vi "create_pb_arrayofarrays_expansion_v2.vi"(0 "Arbitrary Waveform Array of Channels":T2(array[cluster])=[[{"AC Frequency (kHz)"=40.0, " Initial AC Ampl. (p-p/2)"=0.0, "Final AC Ampl."=0.0, "Initial DC Value"=-0.25, "Final DC Value"=0.05, "Constant"=165.3, "Gamma AC"=1.0, "String"="Channel 0 A", "Gamma DC"=1.0}, {"AC Frequency (kHz)"=40.0, " Initial AC Ampl. (p-p/2)"=0.0, "Final AC Ampl."=0.0, "Initial DC Value"=0.0, "Final DC Value"=0.0, "Constant"=165.2, "Gamma AC"=1.0, "String"="Channel 0 B", "Gamma DC"=1.0}, {"AC Frequency (kHz)"=40.0, " Initial AC Ampl. (p-p/2)"=0.0, "Final AC Ampl."=0.0, "Initial DC Value"=0.0, "Final DC Value"=0.0, "Constant"=163.20000000000002, "Gamma AC"=1.0, "String"="Channel 0 C", "Gamma DC"=1.0}], [{"AC Frequency (kHz)"=10.0, " Initial AC Ampl. (p-p/2)"=5.0, "Final AC Ampl."=0.0, "Initial DC Value"=0.2, "Final DC Value"=0.14, "Constant"=0.25, "Gamma AC"=1.0, "String"="Channel 1 A", "Gamma DC"=1.0}, {"AC Frequency (kHz)"=10.0, " Initial AC Ampl. (p-p/2)"=5.0, "Final AC Ampl."=0.0, "Initial DC Value"=0.1, "Final DC Value"=0.1, "Constant"=0.25, "Gamma AC"=1.0, "String"="Channel 1 B", "Gamma DC"=1.0}, {"AC Frequency (kHz)"=10.0, " Initial AC Ampl. (p-p/2)"=0.0, "Final AC Ampl."=0.0, "Initial DC Value"=0.0, "Final DC Value"=0.0, "Constant"=0.25, "Gamma AC"=1.0, "String"="Channel 1 C", "Gamma DC"=1.0}], [{"AC Frequency (kHz)"=10.0, " Initial AC Ampl. (p-p/2)"=0.0, "Final AC Ampl."=0.0, "Initial DC Value"=0.007, "Final DC Value"=0.04, "Constant"=0.0, "Gamma AC"=1.0, "String"="Channel 2 A", "Gamma DC"=1.0}, {"AC Frequency (kHz)"=10.0, " Initial AC Ampl. (p-p/2)"=0.0, "Final AC Ampl."=0.0, "Initial DC Value"=0.5, "Final DC Value"=0.5, "Constant"=0.0, "Gamma AC"=1.0, "String"="Channel 2 B", "Gamma DC"=1.0}, {"AC Frequency (kHz)"=10.0, " Initial AC Ampl. (p-p/2)"=0.0, "Final AC Ampl."=0.0, "Initial DC Value"=0.0, "Final DC Value"=0.0, "Constant"=0.0, "Gamma AC"=1.0, "String"="Channel 2 C", "Gamma DC"=1.0}], [{"AC Frequency (kHz)"=10.0, " Initial AC Ampl. (p-p/2)"=0.0, "Final AC Ampl."=0.0, "Initial DC Value"=1.0, "Final DC Value"=1.0, "Constant"=199.2, "Gamma AC"=1.0, "String"="Channel 3 A", "Gamma DC"=1.0}, {"AC Frequency (kHz)"=10.0, " Initial AC Ampl. (p-p/2)"=0.0, "Final AC Ampl."=0.0, "Initial DC Value"=1.0, "Final DC Value"=1.0, "Constant"=199.2, "Gamma AC"=1.0, "String"="Channel 3 B", "Gamma DC"=1.0}, {"AC Frequency (kHz)"=10.0, " Initial AC Ampl. (p-p/2)"=0.0, "Final AC Ampl."=0.0, "Initial DC Value"=1.0, "Final DC Value"=1.0, "Constant"=199.2, "Gamma AC"=1.0, "String"="Channel 3 C", "Gamma DC"=1.0}], [{"AC Frequency (kHz)"=10.0, " Initial AC Ampl. (p-p/2)"=0.0, "Final AC Ampl."=0.0, "Initial DC Value"=-0.1, "Final DC Value"=-0.04, "Constant"=199.2, "Gamma AC"=1.0, "String"="Channel 4 A", "Gamma DC"=1.0}, {"AC Frequency (kHz)"=10.0, " Initial AC Ampl. (p-p/2)"=0.0, "Final AC Ampl."=0.0, "Initial DC Value"=-0.1, "Final DC Value"=-0.04, "Constant"=199.2, "Gamma AC"=1.0, "String"="Channel 4 B", "Gamma DC"=1.0}, {"AC Frequency (kHz)"=10.0, " Initial AC Ampl. (p-p/2)"=0.0, "Final AC Ampl."=0.0, "Initial DC Value"=-0.1, "Final DC Value"=-0.04, "Constant"=199.2, "Gamma AC"=1.0, "String"="Channel 4 C", "Gamma DC"=1.0}], [{"AC Frequency (kHz)"=10.0, " Initial AC Ampl. (p-p/2)"=0.0, "Final AC Ampl."=0.0, "Initial DC Value"=-0.1, "Final DC Value"=-0.04, "Constant"=199.2, "Gamma AC"=1.0, "String"="Channel 5 A", "Gamma DC"=1.0}, {"AC Frequency (kHz)"=10.0, " Initial AC Ampl. (p-p/2)"=0.0, "Final AC Ampl."=0.0, "Initial DC Value"=-0.1, "Final DC Value"=-0.04, "Constant"=199.2, "Gamma AC"=1.0, "String"="Channel 5 B", "Gamma DC"=1.0}, {"AC Frequency (kHz)"=10.0, " Initial AC Ampl. (p-p/2)"=0.0, "Final AC Ampl."=0.0, "Initial DC Value"=-0.1, "Final DC Value"=-0.04, "Constant"=199.2, "Gamma AC"=1.0, "String"="Channel 5 C", "Gamma DC"=1.0}], [{"AC Frequency (kHz)"=10.0, " Initial AC Ampl. (p-p/2)"=0.0, "Final AC Ampl."=0.0, "Initial DC Value"=-0.1, "Final DC Value"=-0.04, "Constant"=199.2, "Gamma AC"=1.0, "String"="Channel 6 A", "Gamma DC"=1.0}, {"AC Frequency (kHz)"=10.0, " Initial AC Ampl. (p-p/2)"=0.0, "Final AC Ampl."=0.0, "Initial DC Value"=-0.1, "Final DC Value"=-0.04, "Constant"=199.2, "Gamma AC"=1.0, "String"="Channel 6 B", "Gamma DC"=1.0}, {"AC Frequency (kHz)"=10.0, " Initial AC Ampl. (p-p/2)"=0.0, "Final AC Ampl."=0.0, "Initial DC Value"=-0.1, "Final DC Value"=-0.04, "Constant"=199.2, "Gamma AC"=1.0, "String"="Channel 6 C", "Gamma DC"=1.0}], [{"AC Frequency (kHz)"=10.0, " Initial AC Ampl. (p-p/2)"=0.0, "Final AC Ampl."=0.0, "Initial DC Value"=-0.1, "Final DC Value"=-0.04, "Constant"=199.2, "Gamma AC"=1.0, "String"="Channel 7 A", "Gamma DC"=1.0}, {"AC Frequency (kHz)"=10.0, " Initial AC Ampl. (p-p/2)"=0.0, "Final AC Ampl."=0.0, "Initial DC Value"=-0.1, "Final DC Value"=-0.04, "Constant"=199.2, "Gamma AC"=1.0, "String"="Channel 7 B", "Gamma DC"=1.0}, {"AC Frequency (kHz)"=10.0, " Initial AC Ampl. (p-p/2)"=0.0, "Final AC Ampl."=0.0, "Initial DC Value"=-0.1, "Final DC Value"=-0.04, "Constant"=199.2, "Gamma AC"=1.0, "String"="Channel 7 C", "Gamma DC"=1.0}]] {"Gamma DC" format="%.2f"; "Gamma AC" format="%.2f"; "Constant" min=0.0 max=240.0 format="%.3f"; "Final DC Value" format="%.3f"; "Initial DC Value" format="%.3f"; "Final AC Ampl." format="%.3f"; "Initial AC Ampl. (p-p/2)" format="%.3f"; "AC Frequency (kHz)" format="%.2f"}, 2 "Parameters to Change":T9={"PB parameter to change"=0, "Column of\nData to Change\n(0, 1, 2, ....)"=0, "Column of\nDelay to Change\n(0, 1, 2, ....)"=11, "6713 DAC Ch\nto Change"=7, "column for waveform\n(red mot cooling)"=10, "# of PB arrays"=1, "column for waveform\n(dipole trap loading)"=10, "Power\nSupply\nChannel"=1} {"Power\nSupply\nChannel" min=1 max=2; "PB parameter to change" min=0 max=4}, 5 "87Sr Waveform Change Parameters":T6={"Channel to Change"=0, "Interval to Change"=1, "Waveform Parameter\nto Change"=8} {"Waveform Parameter\nto Change" items=["Constant", "Initial DC", "Final DC", "Gamma DC", "AC Frequency", "Initial AC", "Gamma AC", "Final AC", "Interval Length"]; "Interval to Change" items=["A", "B", "C", "D"]}, 7 "87Sr Interval Lengths (ms)":dbl[](array[numeric])=[55.0, 45.0, 1.0] format="%.3f", 9 "87Sr Intervals: ON or OFF?":bool[](array[boolean])=[TRUE, FALSE, FALSE], 11 "Generated Array":T7={"Step Size"=-0.03, "Use generated\nDAC array values?"=FALSE, "Number of DAC Array\nValues to Generate"=67, "Initial Value for DAC"=[1.0]} {"Initial Value for DAC" format="%.2f"; "Step Size" format="%.4f"}, 12 "Logarithmic Array":T5={"Initial Value"=1, "Fineness Factor"=1, "Number of Values"=10, "Generate Logarithmic\nArray?"=FALSE}, 13 "Lattice Waveform Array of Channels":T2(array[cluster])=[[{"AC Frequency (kHz)"=40.0, " Initial AC Ampl. (p-p/2)"=0.0, "Final AC Ampl."=0.0, "Initial DC Value"=-0.25, "Final DC Value"=0.05, "Constant"=165.3, "Gamma AC"=1.0, "String"="Channel 0 A", "Gamma DC"=1.0}, {"AC Frequency (kHz)"=40.0, " Initial AC Ampl. (p-p/2)"=0.0, "Final AC Ampl."=0.0, "Initial DC Value"=0.0, "Final DC Value"=0.0, "Constant"=165.2, "Gamma AC"=1.0, "String"="Channel 0 B", "Gamma DC"=1.0}, {"AC Frequency (kHz)"=40.0, " Initial AC Ampl. (p-p/2)"=0.0, "Final AC Ampl."=0.0, "Initial DC Value"=0.0, "Final DC Value"=0.0, "Constant"=163.20000000000002, "Gamma AC"=1.0, "String"="Channel 0 C", "Gamma DC"=1.0}], [{"AC Frequency (kHz)"=10.0, " Initial AC Ampl. (p-p/2)"=5.0, "Final AC Ampl."=0.0, "Initial DC Value"=0.2, "Final DC Value"=0.14, "Constant"=0.25, "Gamma AC"=1.0, "String"="Channel 1 A", "Gamma DC"=1.0}, {"AC Frequency (kHz)"=10.0, " Initial AC Ampl. (p-p/2)"=5.0, "Final AC Ampl."=0.0, "Initial DC Value"=0.1, "Final DC Value"=0.1, "Constant"=0.25, "Gamma AC"=1.0, "String"="Channel 1 B", "Gamma DC"=1.0}, {"AC Frequency (kHz)"=10.0, " Initial AC Ampl. (p-p/2)"=0.0, "Final AC Ampl."=0.0, "Initial DC Value"=0.0, "Final DC Value"=0.0, "Constant"=0.25, "Gamma AC"=1.0, "String"="Channel 1 C", "Gamma DC"=1.0}], [{"AC Frequency (kHz)"=10.0, " Initial AC Ampl. (p-p/2)"=0.0, "Final AC Ampl."=0.0, "Initial DC Value"=0.007, "Final DC Value"=0.04, "Constant"=0.0, "Gamma AC"=1.0, "String"="Channel 2 A", "Gamma DC"=1.0}, {"AC Frequency (kHz)"=10.0, " Initial AC Ampl. (p-p/2)"=0.0, "Final AC Ampl."=0.0, "Initial DC Value"=0.5, "Final DC Value"=0.5, "Constant"=0.0, "Gamma AC"=1.0, "String"="Channel 2 B", "Gamma DC"=1.0}, {"AC Frequency (kHz)"=10.0, " Initial AC Ampl. (p-p/2)"=0.0, "Final AC Ampl."=0.0, "Initial DC Value"=0.0, "Final DC Value"=0.0, "Constant"=0.0, "Gamma AC"=1.0, "String"="Channel 2 C", "Gamma DC"=1.0}], [{"AC Frequency (kHz)"=10.0, " Initial AC Ampl. (p-p/2)"=0.0, "Final AC Ampl."=0.0, "Initial DC Value"=1.0, "Final DC Value"=1.0, "Constant"=199.2, "Gamma AC"=1.0, "String"="Channel 3 A", "Gamma DC"=1.0}, {"AC Frequency (kHz)"=10.0, " Initial AC Ampl. (p-p/2)"=0.0, "Final AC Ampl."=0.0, "Initial DC Value"=1.0, "Final DC Value"=1.0, "Constant"=199.2, "Gamma AC"=1.0, "String"="Channel 3 B", "Gamma DC"=1.0}, {"AC Frequency (kHz)"=10.0, " Initial AC Ampl. (p-p/2)"=0.0, "Final AC Ampl."=0.0, "Initial DC Value"=1.0, "Final DC Value"=1.0, "Constant"=199.2, "Gamma AC"=1.0, "String"="Channel 3 C", "Gamma DC"=1.0}], [{"AC Frequency (kHz)"=10.0, " Initial AC Ampl. (p-p/2)"=0.0, "Final AC Ampl."=0.0, "Initial DC Value"=-0.1, "Final DC Value"=-0.04, "Constant"=199.2, "Gamma AC"=1.0, "String"="Channel 4 A", "Gamma DC"=1.0}, {"AC Frequency (kHz)"=10.0, " Initial AC Ampl. (p-p/2)"=0.0, "Final AC Ampl."=0.0, "Initial DC Value"=-0.1, "Final DC Value"=-0.04, "Constant"=199.2, "Gamma AC"=1.0, "String"="Channel 4 B", "Gamma DC"=1.0}, {"AC Frequency (kHz)"=10.0, " Initial AC Ampl. (p-p/2)"=0.0, "Final AC Ampl."=0.0, "Initial DC Value"=-0.1, "Final DC Value"=-0.04, "Constant"=199.2, "Gamma AC"=1.0, "String"="Channel 4 C", "Gamma DC"=1.0}], [{"AC Frequency (kHz)"=10.0, " Initial AC Ampl. (p-p/2)"=0.0, "Final AC Ampl."=0.0, "Initial DC Value"=-0.1, "Final DC Value"=-0.04, "Constant"=199.2, "Gamma AC"=1.0, "String"="Channel 5 A", "Gamma DC"=1.0}, {"AC Frequency (kHz)"=10.0, " Initial AC Ampl. (p-p/2)"=0.0, "Final AC Ampl."=0.0, "Initial DC Value"=-0.1, "Final DC Value"=-0.04, "Constant"=199.2, "Gamma AC"=1.0, "String"="Channel 5 B", "Gamma DC"=1.0}, {"AC Frequency (kHz)"=10.0, " Initial AC Ampl. (p-p/2)"=0.0, "Final AC Ampl."=0.0, "Initial DC Value"=-0.1, "Final DC Value"=-0.04, "Constant"=199.2, "Gamma AC"=1.0, "String"="Channel 5 C", "Gamma DC"=1.0}], [{"AC Frequency (kHz)"=10.0, " Initial AC Ampl. (p-p/2)"=0.0, "Final AC Ampl."=0.0, "Initial DC Value"=-0.1, "Final DC Value"=-0.04, "Constant"=199.2, "Gamma AC"=1.0, "String"="Channel 6 A", "Gamma DC"=1.0}, {"AC Frequency (kHz)"=10.0, " Initial AC Ampl. (p-p/2)"=0.0, "Final AC Ampl."=0.0, "Initial DC Value"=-0.1, "Final DC Value"=-0.04, "Constant"=199.2, "Gamma AC"=1.0, "String"="Channel 6 B", "Gamma DC"=1.0}, {"AC Frequency (kHz)"=10.0, " Initial AC Ampl. (p-p/2)"=0.0, "Final AC Ampl."=0.0, "Initial DC Value"=-0.1, "Final DC Value"=-0.04, "Constant"=199.2, "Gamma AC"=1.0, "String"="Channel 6 C", "Gamma DC"=1.0}], [{"AC Frequency (kHz)"=10.0, " Initial AC Ampl. (p-p/2)"=0.0, "Final AC Ampl."=0.0, "Initial DC Value"=-0.1, "Final DC Value"=-0.04, "Constant"=199.2, "Gamma AC"=1.0, "String"="Channel 7 A", "Gamma DC"=1.0}, {"AC Frequency (kHz)"=10.0, " Initial AC Ampl. (p-p/2)"=0.0, "Final AC Ampl."=0.0, "Initial DC Value"=-0.1, "Final DC Value"=-0.04, "Constant"=199.2, "Gamma AC"=1.0, "String"="Channel 7 B", "Gamma DC"=1.0}, {"AC Frequency (kHz)"=10.0, " Initial AC Ampl. (p-p/2)"=0.0, "Final AC Ampl."=0.0, "Initial DC Value"=-0.1, "Final DC Value"=-0.04, "Constant"=199.2, "Gamma AC"=1.0, "String"="Channel 7 C", "Gamma DC"=1.0}]] {"Gamma DC" format="%.2f"; "Gamma AC" format="%.2f"; "Constant" min=0.0 max=240.0 format="%.3f"; "Final DC Value" format="%.3f"; "Initial DC Value" format="%.3f"; "Final AC Ampl." format="%.3f"; "Initial AC Ampl. (p-p/2)" format="%.3f"; "AC Frequency (kHz)" format="%.2f"}) -> (1 "changed\nquantity":dbl[](array[numeric]), 4 "Lattice Waveform \nArray of Channels":T1(array[cluster]), 6 "87 Sr ArbWaveform \nArray of Channels":T1(array[cluster]), 8 "87Sr ArbWaveform Interval Lengths":dbl[][](array[numeric]), 10 "Generated\nDAC Array":dbl[](array[numeric])=[1.0, 0.97, 0.94, 0.9099999999999999, 0.8799999999999999, 0.8499999999999999, 0.8199999999999998, 0.7899999999999998, 0.7599999999999998, 0.7299999999999998, 0.6999999999999997, 0.6699999999999997, 0.6399999999999997, 0.6099999999999997, 0.5799999999999996, 0.5499999999999996, 0.5199999999999996, 0.48999999999999955, 0.4599999999999995, 0.4299999999999995, 0.39999999999999947, 0.36999999999999944, 0.3399999999999994, 0.3099999999999994, 0.27999999999999936, 0.24999999999999936, 0.21999999999999936, 0.18999999999999936, 0.15999999999999936, 0.12999999999999937, 0.09999999999999937, 0.06999999999999937, 0.03999999999999937, 0.00999999999999937, -0.02000000000000063, -0.05000000000000063, -0.08000000000000063, -0.11000000000000063, -0.14000000000000062, -0.17000000000000062, -0.20000000000000062, -0.23000000000000062, -0.2600000000000006, -0.2900000000000006, -0.3200000000000006, -0.35000000000000064, -0.38000000000000067, -0.4100000000000007, -0.4400000000000007, -0.47000000000000075, -0.5000000000000008, -0.5300000000000008, -0.5600000000000008, -0.5900000000000009, -0.6200000000000009, -0.6500000000000009, -0.6800000000000009, -0.710000000000001, -0.740000000000001, -0.770000000000001, -0.800000000000001, -0.8300000000000011, -0.8600000000000011, -0.8900000000000011, -0.9200000000000012, -0.9500000000000012, -0.9800000000000012, -1.0100000000000011] format="%.4f", 15 "output params to change":T8)   [LabVIEW 2013]
panel:
  in  "Case Constant\n(See Context Help)":bool
  out "PB Array of Arrays":T3(array[cluster])
  in  "PulseBlaster Array of Arrays":T4(array[cluster])=[{"Data Field"=0, "Delay"=0.005, "OP code"=8, "Output Bits"=[FALSE, TRUE, FALSE, FALSE, FALSE, FALSE, FALSE, FALSE, FALSE, FALSE, FALSE, FALSE, TRUE, FALSE, FALSE, FALSE, FALSE, FALSE, FALSE, FALSE, FALSE, FALSE, FALSE, FALSE], "String"="cool mot coils"}, {"Data Field"=300, "Delay"=0.000999, "OP code"=2, "Output Bits"=[TRUE, TRUE, TRUE, TRUE, FALSE, FALSE, TRUE, FALSE, FALSE, TRUE, FALSE, FALSE, TRUE, TRUE, FALSE, TRUE, TRUE, FALSE, FALSE, FALSE, FALSE, FALSE, FALSE, FALSE], "String"="mot load loop"}, {"Data Field"=1, "Delay"=1e-06, "OP code"=3, "Output Bits"=[TRUE, TRUE, TRUE, TRUE, FALSE, FALSE, TRUE, FALSE, FALSE, TRUE, FALSE, FALSE, TRUE, TRUE, FALSE, TRUE, TRUE, FALSE, FALSE, FALSE, FALSE, FALSE, FALSE, FALSE, FALSE], "String"=""}, {"Data Field"=0, "Delay"=0.001, "OP code"=0, "Output Bits"=[TRUE, TRUE, TRUE, TRUE, FALSE, FALSE, TRUE, FALSE, FALSE, TRUE, FALSE, FALSE, TRUE, TRUE, FALSE, TRUE, TRUE, FALSE, FALSE, FALSE, FALSE, FALSE, FALSE, FALSE], "String"=""}, {"Data Field"=2, "Delay"=0.000999, "OP code"=2, "Output Bits"=[TRUE, TRUE, TRUE, TRUE, FALSE, FALSE, TRUE, FALSE, FALSE, TRUE, FALSE, FALSE, TRUE, TRUE, FALSE, TRUE, TRUE, FALSE, FALSE, FALSE, FALSE, FALSE, FALSE, FALSE], "String"="mot decay loop"}, {"Data Field"=4, "Delay"=1e-06, "OP code"=3, "Output Bits"=[TRUE, TRUE, TRUE, TRUE, FALSE, FALSE, TRUE, FALSE, FALSE, TRUE, FALSE, FALSE, TRUE, TRUE, FALSE, TRUE, TRUE, FALSE, FALSE, FALSE, FALSE, FALSE, FALSE, FALSE], "String"=""}, {"Data Field"=0, "Delay"=0.000908, "OP code"=0, "Output Bits"=[TRUE, TRUE, TRUE, TRUE, FALSE, FALSE, TRUE, FALSE, FALSE, TRUE, FALSE, FALSE, TRUE, TRUE, FALSE, TRUE, TRUE, FALSE, FALSE, FALSE, FALSE, FALSE, FALSE, FALSE], "String"=""}, {"Data Field"=0, "Delay"=0.00865, "OP code"=0, "Output Bits"=[TRUE, TRUE, TRUE, TRUE, FALSE, FALSE, TRUE, FALSE, FALSE, TRUE, FALSE, FALSE, TRUE, TRUE, FALSE, TRUE, TRUE, FALSE, FALSE, FALSE, FALSE, FALSE, FALSE, FALSE], "String"=""}, {"Data Field"=0, "Delay"=0.004, "OP code"=0, "Output Bits"=[TRUE, TRUE, FALSE, TRUE, FALSE, FALSE, TRUE, FALSE, FALSE, TRUE, FALSE, FALSE, TRUE, TRUE, FALSE, TRUE, TRUE, FALSE, FALSE, FALSE, FALSE, FALSE, FALSE, FALSE], "String"=""}, {"Data Field"=0, "Delay"=0.0045, "OP code"=0, "Output Bits"=[TRUE, TRUE, FALSE, TRUE, FALSE, FALSE, TRUE, FALSE, FALSE, TRUE, FALSE, FALSE, TRUE, FALSE, FALSE, FALSE, TRUE, FALSE, FALSE, FALSE, FALSE, FALSE, FALSE, FALSE], "String"="Blue MOT Cooling Time"}, {"Data Field"=0, "Delay"=0.05, "OP code"=0, "Output Bits"=[FALSE, TRUE, FALSE, FALSE, FALSE, FALSE, FALSE, FALSE, FALSE, TRUE, TRUE, FALSE, TRUE, FALSE, FALSE, FALSE, FALSE, FALSE, FALSE, FALSE, FALSE, FALSE, FALSE, FALSE], "String"="Red MOT Cooling Time =="}, {"Data Field"=0, "Delay"=0.01, "OP code"=0, "Output Bits"=[FALSE, TRUE, FALSE, FALSE, FALSE, FALSE, FALSE, FALSE, FALSE, FALSE, FALSE, FALSE, FALSE, FALSE, FALSE, FALSE, FALSE, FALSE, FALSE, FALSE, FALSE, FALSE, FALSE, FALSE], "String"="PAS Beam with RED MOT            DELAY TIME BEFORE INTERAC"}, {"Data Field"=0, "Delay"=0.005, "OP code"=0, "Output Bits"=[FALSE, TRUE, FALSE, FALSE, FALSE, FALSE, FALSE, FALSE, FALSE, FALSE, FALSE, FALSE, FALSE, FALSE, FALSE, FALSE, TRUE, FALSE, FALSE, FALSE, FALSE, FALSE, FALSE, FALSE], "String"="image 12 delay (150n=90ndelay) INTERAC TIME"}, {"Data Field"=0, "Delay"=5e-05, "OP code"=0, "Output Bits"=[FALSE, TRUE, FALSE, FALSE, FALSE, FALSE, FALSE, FALSE, FALSE, FALSE, FALSE, FALSE, FALSE, FALSE, FALSE, FALSE, TRUE, TRUE, FALSE, FALSE, FALSE, FALSE, FALSE, FALSE], "String"="image beam on"}, {"Data Field"=0, "Delay"=0.0002, "OP code"=0, "Output Bits"=[FALSE, FALSE, FALSE, FALSE, FALSE, TRUE, FALSE, FALSE, FALSE, FALSE, FALSE, FALSE, FALSE, FALSE, FALSE, FALSE, TRUE, TRUE, FALSE, FALSE, FALSE, FALSE, FALSE, FALSE], "String"="camera minimum exposure time"}, {"Data Field"=0, "Delay"=0.07, "OP code"=0, "Output Bits"=[FALSE, FALSE, FALSE, FALSE, FALSE, FALSE, FALSE, FALSE, FALSE, FALSE, FALSE, FALSE, FALSE, FALSE, FALSE, FALSE, FALSE, TRUE, FALSE, FALSE, FALSE, FALSE, FALSE, FALSE], "String"="PixelFly Readout 1"}, {"Data Field"=0, "Delay"=0.005, "OP code"=0, "Output Bits"=[FALSE, FALSE, FALSE, FALSE, FALSE, FALSE, FALSE, FALSE, FALSE, FALSE, FALSE, FALSE, FALSE, FALSE, FALSE, FALSE, TRUE, TRUE, FALSE, FALSE, FALSE, FALSE, FALSE, FALSE], "String"="shutter opening time"}, {"Data Field"=0, "Delay"=0.0002, "OP code"=0, "Output Bits"=[FALSE, FALSE, FALSE, FALSE, FALSE, TRUE, FALSE, FALSE, FALSE, FALSE, FALSE, FALSE, FALSE, FALSE, FALSE, FALSE, TRUE, TRUE, FALSE, FALSE, FALSE, FALSE, FALSE, FALSE], "String"="Pixelfly exposure 2"}, {"Data Field"=0, "Delay"=0.07, "OP code"=0, "Output Bits"=[FALSE, FALSE, FALSE, FALSE, FALSE, FALSE, FALSE, FALSE, FALSE, FALSE, FALSE, FALSE, FALSE, FALSE, FALSE, FALSE, FALSE, FALSE, FALSE, FALSE, FALSE, FALSE, FALSE, FALSE], "String"="PixelFly readout 2"}, {"Data Field"=0, "Delay"=0.001, "OP code"=6, "Output Bits"=[FALSE, TRUE, TRUE, TRUE, FALSE, FALSE, FALSE, FALSE, FALSE, FALSE, FALSE, FALSE, TRUE, TRUE, FALSE, TRUE, FALSE, FALSE, FALSE, FALSE, FALSE, FALSE, FALSE, FALSE], "String"=""}] {"OP code" items=["Continue", "Stop", "Loop", "End Loop", "Jump", "Return", "Go To", "Long Delay", "Wait"]; "Delay" format="%.3p"}
  in  "Manual Array":dbl[](array[numeric])=[0.05, 0.1, 0.15, 0.2, 0.25, 0.3, 0.35, 0.4, 0.45, 0.5, 9.6, 0.24, 0.26, 5.28, 0.3, 0.32, 0.34, 0.36, 0.38, 0.4, 5.0, 5.2, 5.4, 5.6, 5.8, 6.0, 6.2, 6.4, 6.6, 6.8, 7.0, 7.199999999999999, 7.4, 7.6, 7.800000000000001, 9.0, 6.8, 7.2, 7.6, 8.0, 8.4, 8.8, 9.0, 9.2, 9.4, 9.6, 9.8, 10.0, 0.4, 0.2, 0.0001, 0.0001, 0.0001, 0.0001, 0.0001, 0.0001, 0.0001, 0.0001, 0.0001, 0.0001, 0.0001, 0.0001, 0.0001, 0.0001, 0.0001, 0.0001, 0.0001, 0.0001, 0.0001, 0.0001, 0.0001, 0.0001, 0.0001, 0.0001, 0.0001, 0.0001, 0.0001, 0.0001, 0.0001, 0.0001, 0.0001, 0.0001, 0.0001, 0.0001, 0.0001, 0.0001, 0.0001, 0.0001, 0.0001, 0.0001, 0.0001, 0.0001, 0.0001, 0.0001, 0.0001, 0.0001, 0.0001, 0.0001, 0.0001, 0.0001, 0.0001, 0.0001, 0.0001, 0.0001, 0.0001, 0.0001, 0.0001, 0.0001, 0.0001, 0.0001, 0.0001, 0.0001, 0.0001, 0.0001, 0.0001, 0.0001, 0.0001, 0.0001, 0.0001, 0.0001, 0.0001, 0.0001, 0.0001, 0.0001, 0.0001, 0.0001, 0.0001, 0.0001, 0.0001, 0.0001, 0.0001, 0.0001, 0.0001, 0.0001, 0.0001, 0.0001, 0.0001, 0.0001, 0.0001, 0.0001, 0.0001, 0.0001, 0.0001, 0.0001, 0.0001, 0.0001, 0.0, 0.0, 0.0, 0.0, 0.0, 0.0, 0.0, 0.0, 0.0, 0.0, 0.0, 0.0, 0.0, 0.0, 0.0, 0.0, 0.0, 0.0, 0.0, 0.0, 0.0, 0.0, 0.0, 0.0, 0.0, 0.0, 0.0, 0.0, 0.0, 0.0, 0.0, 0.0, 0.0, 0.0, 0.0, 0.0, 0.0, 0.0, 0.0, 0.0, 0.0, 0.0, 0.0, 0.0, 0.0, 0.0, 0.0, 0.0, 0.0, 0.0, 0.0, 0.0, 0.0, 0.0, 0.0, 0.0, 0.0, 0.0, 0.0, 0.0, 0.0, 0.0, 0.0, 0.0, 0.0, 0.0, 0.0, 0.0, 0.0, 0.0, 0.0, 0.0, 0.0, 0.0, 0.0, 0.0, 0.0, 0.0, 0.0, 0.0, 0.0, 0.0, 0.0, 0.0, 0.0, 0.0, 0.0, 0.0, 0.0, 0.0, 0.0, 0.0, 0.0, 0.0, 0.0, 0.0, 0.0, 0.0, 0.0, 0.0, 0.0, 0.0, 0.0, 0.0, 0.0, 0.0, 0.0, 0.0, 0.0, 0.0, 0.0, 0.0, 0.0, 0.0, 0.0, 0.0, 0.0, 0.0, 0.0, 0.0, 0.0, 0.0, 0.0, 0.0, 0.0, 0.0, 0.0, 0.0, 0.0, 0.0, 0.0, 0.0, 0.0, 0.0, 0.0, 0.0, 0.0, 0.0, 0.0, 0.0, 0.0, 0.0, 0.0, 0.0, 0.0, 0.0, 0.0, 0.0, 0.0, 0.0, 0.0, 0.0, 0.0, 0.0, 0.0, 0.0, 0.0, 0.0, 0.0, 0.0, 0.0, 0.0, 0.0, 0.0, 0.0, 0.0, 0.0, 0.0, 0.0, 0.0, 0.0, 0.0, 0.0, 0.0, 0.0, 0.0, 0.0, 0.0, 0.0, 0.0, 0.0, 0.0, 0.0, 0.0, 0.0, 0.0, 0.0, 0.0, 0.0, 0.0, 0.0, 0.0, 0.0, 0.0, 0.0, 0.0, 0.0, 0.0, 0.0, 0.0, 0.0, 0.0, 0.0, 0.0, 0.0, 0.0, 0.0, 0.0, 0.0, 0.0, 0.0, 0.0, 0.0, 0.0, 0.0, 0.0, 0.0, 0.0, 0.0, 0.0, 0.0, 0.0, 0.0, 0.0, 0.0, 0.0, 0.0, 0.0, 0.0, 0.0, 0.0, 0.0, 0.0, 0.0, 0.0, 0.0, 0.0, 0.0, 0.0, 0.0, 0.0, 0.0, 0.0, 0.0, 0.0, 0.0, 0.0, 0.0, 0.0, 0.0, 0.0, 0.0, 0.0, 0.0, 0.0, 0.0, 0.0, 0.0, 0.0, 0.0, 0.0, 0.0, 0.0, 0.0, 0.0, 0.0, 0.0, 0.0, 0.0, 0.0, 0.0, 0.0, 0.0, 0.0, 0.0, 0.0, 0.0, 0.0, 0.0, 0.0, 0.0, 0.0, 0.0, 0.0, 0.0, 0.0, 0.0, 0.0, 0.0, 0.0, 0.0, 0.0, 0.0, 0.0, 0.0, 0.0, 0.0, 0.0, 0.0, 0.0, 0.0, 0.0, 0.0, 0.0, 0.0, 0.0, 0.0, 0.0, 0.0, 0.0, 0.0, 0.0, 0.0, 0.0, 0.0, 0.0, 0.0, 0.0, 0.0, 0.0, 0.0, 0.0, 0.0, 0.0, 0.0, 0.0, 0.0, 0.0, 0.0, 0.0, 0.0, 0.0, 0.0, 0.0, 0.0, 0.0, 0.0, 0.0, 0.0, 0.0, 0.0, 0.0, 0.0, 0.0, 0.0, 0.0, 0.0, 0.0, 0.0, 0.0, 0.0, 0.0, 0.0, 0.0, 0.0] caption="Manual array" format="%.3f"
  out "red mot cooling time":dbl[](array[numeric])
  # "(smaller makes\nblue)"
  # "(smaller makes\nblue)"
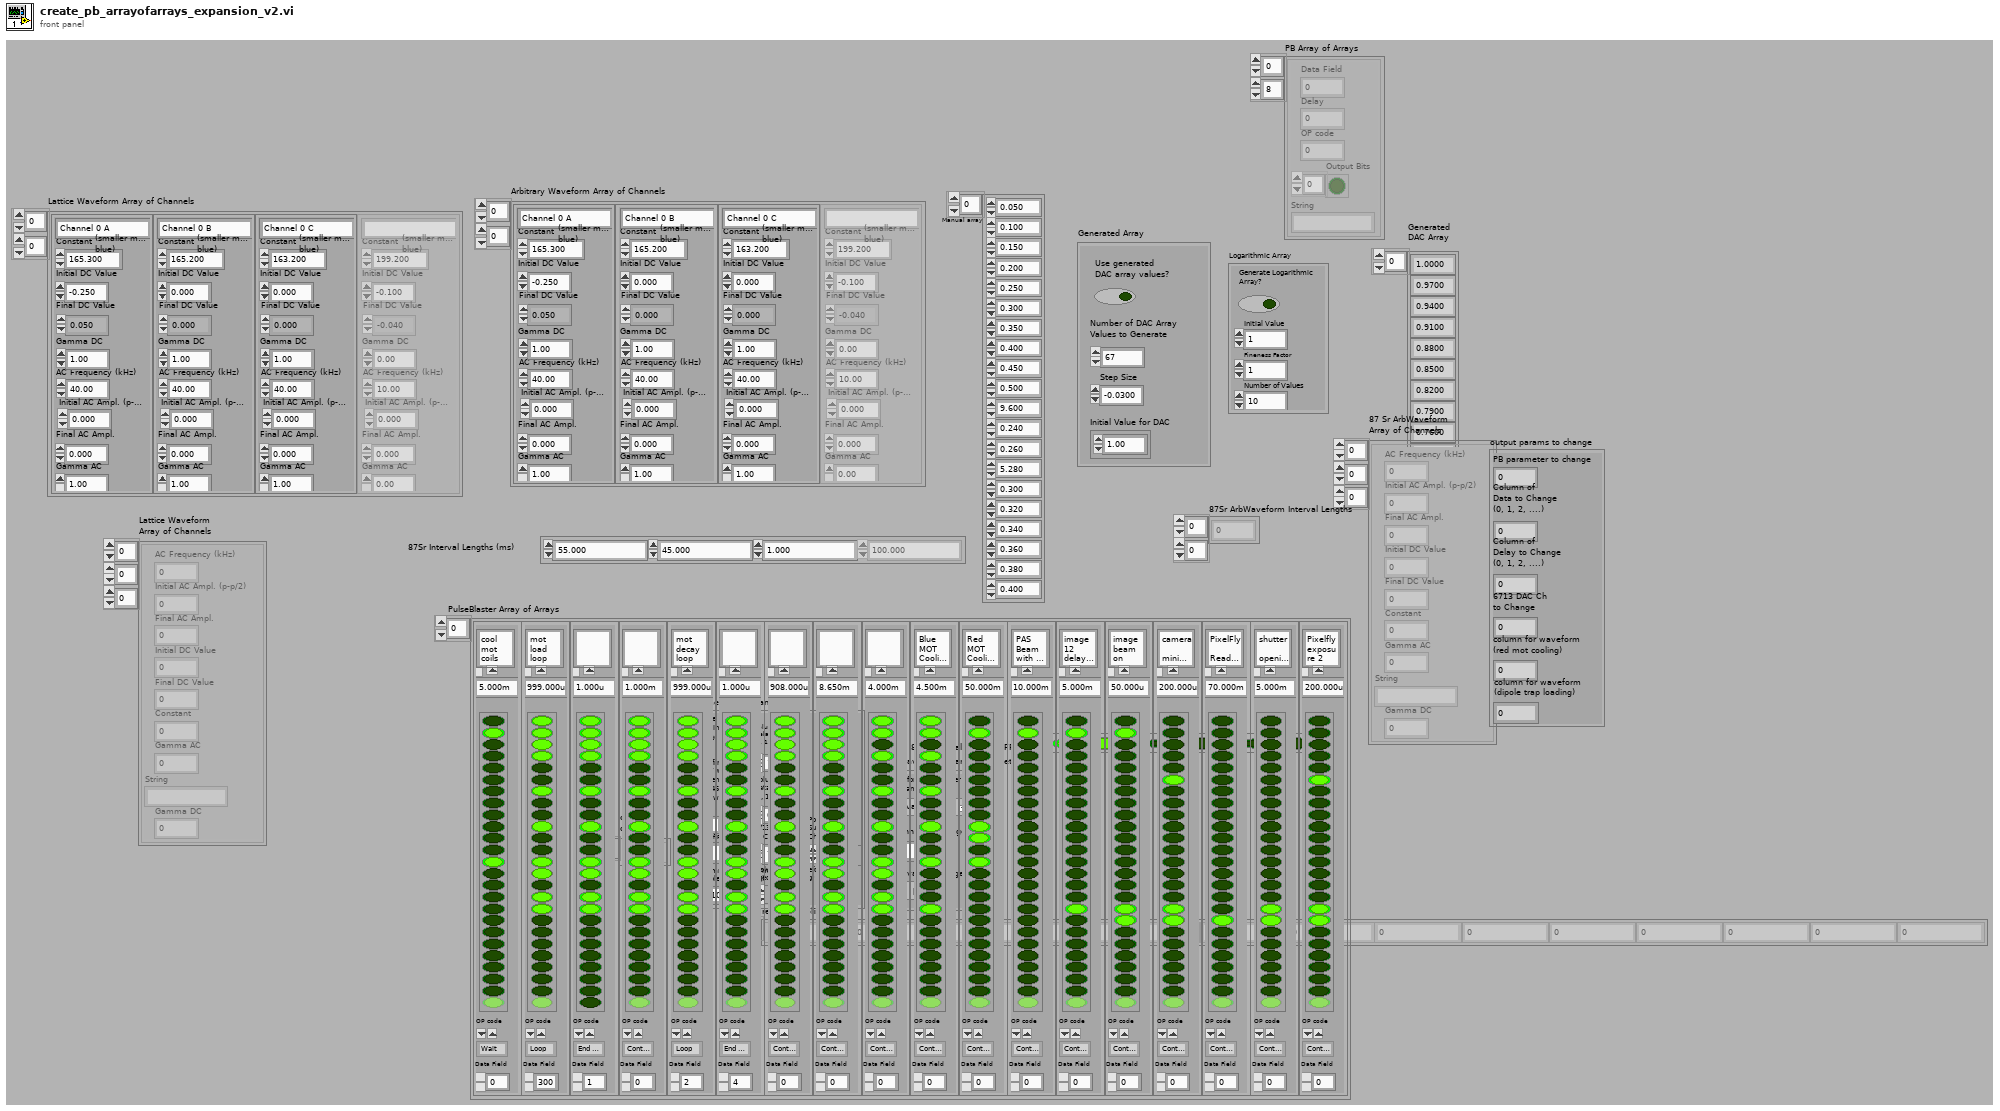
[diagram p1: front panel]
types:
  T1 = cluster{"AC Frequency (kHz)":dbl, "Initial AC Ampl. (p-p/2)":dbl, "Final AC Ampl.":dbl, "Initial DC Value":dbl, "Final DC Value":dbl, "Constant":dbl, "Gamma AC":dbl, "String":string, "Gamma DC":dbl}[][][]
  T2 = cluster{"AC Frequency (kHz)":dbl, " Initial AC Ampl. (p-p/2)":dbl, "Final AC Ampl.":dbl, "Initial DC Value":dbl, "Final DC Value":dbl, "Constant":dbl, "Gamma AC":dbl, "String":string, "Gamma DC":dbl}[][]
  T3 = cluster{"Data Field":u32, "Delay":dbl, "OP code":u8, "Output Bits":bool[], "String":string}[][]
  T4 = cluster{"Data Field":u32, "Delay":dbl, "OP code":u8, "Output Bits":bool[], "String":string}[]
  T5 = cluster{"Initial Value":i32, "Fineness Factor":i32, "Number of Values":i32, "Generate Logarithmic\nArray?":bool}
  T6 = cluster{"Channel to Change":i8, "Interval to Change":i8, "Waveform Parameter\nto Change":u16}
  T7 = cluster{"Step Size":dbl, "Use generated\nDAC array values?":bool, "Number of DAC Array\nValues to Generate":i32, "Initial Value for DAC":dbl[]}
  T8 = cluster{"PB parameter to change":i8, "Column of\nData to Change\n(0, 1, 2, ....)":i32, "Column of\nDelay to Change\n(0, 1, 2, ....)":i32, "6713 DAC Ch\nto Change":i32, "column for waveform\n(red mot cooling)":i32, "column for waveform\n(dipole trap loading)":i32}
  T9 = cluster{"PB parameter to change":i8, "Column of\nData to Change\n(0, 1, 2, ....)":i32, "Column of\nDelay to Change\n(0, 1, 2, ....)":i32, "6713 DAC Ch\nto Change":i32, "column for waveform\n(red mot cooling)":i32, "# of PB arrays":i32, "column for waveform\n(dipole trap loading)":i32, "Power\nSupply\nChannel":i32}
  T10 = cluster{"AC Frequency (kHz)":dbl, " Initial AC Ampl. (p-p/2)":dbl, "Final AC Ampl.":dbl, "Initial DC Value":dbl, "Final DC Value":dbl, "Constant":dbl, "Gamma AC":dbl, "String":string, "Gamma DC":dbl}
  T11 = cluster{"Data Field":u32, "Delay":dbl, "OP code":u8, "Output Bits":bool[], "String":string}
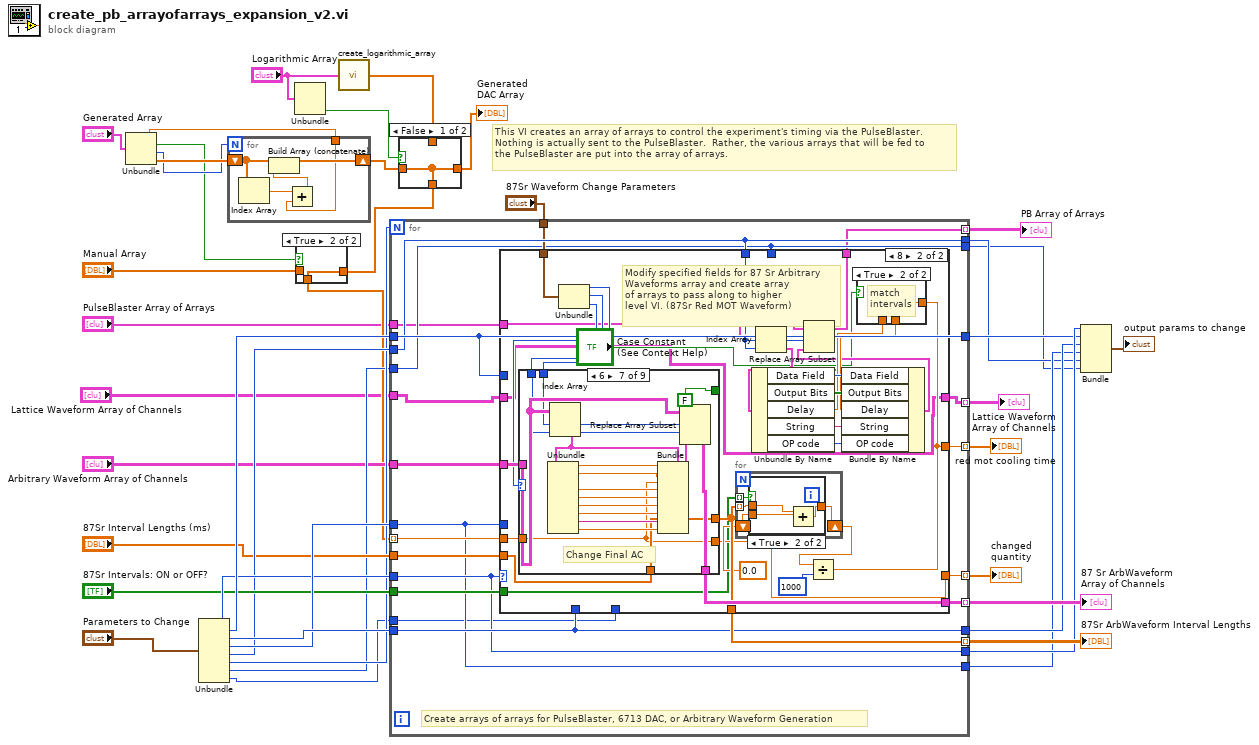
[diagram p0: block diagram]
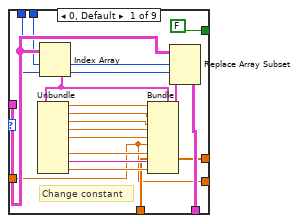
[diagram p7: hidden frame]
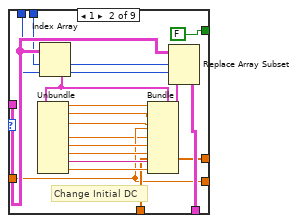
[diagram p8: hidden frame]
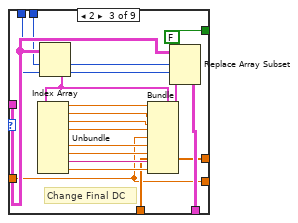
[diagram p9: hidden frame]
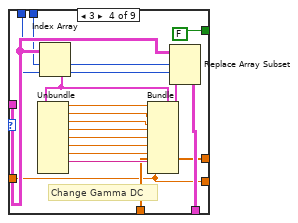
[diagram p10: hidden frame]
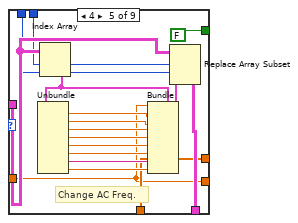
[diagram p11: hidden frame]
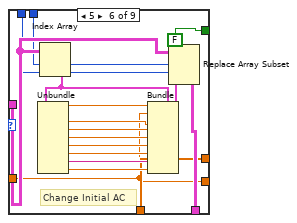
[diagram p12: hidden frame]
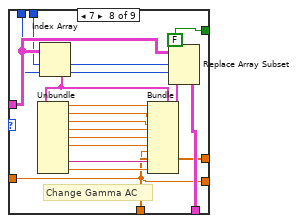
[diagram p13: hidden frame]
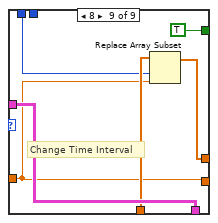
[diagram p14: hidden frame]
diagram:
  # "This VI creates an array of arrays to control the experiment's timing via the PulseBlaster.\nNothing is actually sent to the PulseBlaster.  Rather, the various arrays that will be fed to\nthe PulseBlaster are put into the array of arrays."
  n1 = Unbundle("Generated Array") -> ("Step Size"=w23:dbl, "Use generated\nDAC array values?"=w5:bool, "Number of DAC Array\nValues to Generate"=w24:i32, "Initial Value for DAC"=w25:dbl[])
  n2 = Unbundle("Parameters to Change") -> ("PB parameter to change"=w35:i8, "Column of\nData to Change\n(0, 1, 2, ....)"=w36:i32, "Column of\nDelay to Change\n(0, 1, 2, ....)"=w38:i32, "6713 DAC Ch\nto Change"=w37:i32, "column for waveform\n(red mot cooling)"=w29:i32, "# of PB arrays"=w19:i32, "column for waveform\n(dipole trap loading)"=w17:i32, "Power\nSupply\nChannel"=w15:i32)
  n3 = for {
    N: w24 -> [_]
    shift-right: [w47] -> w11
    shift-left: w25 -> [w46]
    tunnel: w23 -> [w42]
    i -> [w45]
    n4 = Index Array(array=w46, index=w45) -> (element=w44:dbl)
    n5 = Add(x=w44, y=w42) -> (x+y=w43:dbl)
    n6 = Build Array (concatenate)(w46, w43) -> (w47:dbl[])
  }
  n7 = Unbundle("Logarithmic Array") -> ("Generate Logarithmic\nArray?"=w12:bool)  [unwired: 3 out]
  n8 = call "create_logarithmic_array.vi"("Logarithmic Array"="Logarithmic Array") -> ("Generated Log Array"=w10:dbl[])
  n9 = case shown="False" w12 {
    tunnel: [w48 w49] -> w13
    tunnel: w11 -> [w48 _]
    tunnel: w10 -> [_ w49]
    tunnel: [w48 w49] -> w9
    frame False {
    }
    frame True {
    }
  }
  "Generated\nDAC Array" <- w13
  n10 = case shown="True" w5 {
    tunnel: w9 -> [_ w51]
    tunnel: "Manual Array" -> [w50 _]
    tunnel: [w50 w51] -> w6
    frame False {
    }
    frame True {
    }
  }
  n11 = for {
    N: w19 -> [_]
    tunnel: [w62] -> w32
    tunnel: w6 -> [w71] mode=indexing
    tunnel: "87Sr Intervals: ON or OFF?" -> [w70]
    tunnel: [w69] -> w41 mode=indexing
    tunnel: [w68] -> w40 mode=indexing
    tunnel: "Arbitrary Waveform Array of Channels" -> [w67]
    tunnel: w38 -> [w65]
    tunnel: w37 -> [w63]
    tunnel: w36 -> [w62]
    tunnel: w35 -> [w64]
    tunnel: "87Sr Interval Lengths (ms)" -> [w66]
    tunnel: [w65] -> w31
    tunnel: [w64] -> w33
    tunnel: [w63] -> w30
    tunnel: w29 -> [w61]
    tunnel: [w61] -> w28
    tunnel: [w60] -> w22 mode=indexing
    tunnel: [w59] -> w20 mode=indexing
    tunnel: "87Sr Waveform Change Parameters" -> [w58]
    tunnel: w17 -> [w57]
    tunnel: [w57] -> w16
    tunnel: w15 -> [w56]
    tunnel: "PulseBlaster Array of Arrays" -> [w55]
    tunnel: [w54] -> w3 mode=indexing
    tunnel: "Lattice Waveform Array of Channels" -> [w53]
    tunnel: [w52] -> w1 mode=indexing
    # "Create arrays of arrays for PulseBlaster, 6713 DAC, or Arbitrary Waveform Generation"
    n12 = case shown="8" w64 {
      tunnel: w65 -> [_ _]
      tunnel: w63 -> [_ _]
      tunnel: w61 -> [_ w88]
      tunnel: w67 -> [w75 w102]
      tunnel: w71 -> [_ w101]
      tunnel: [w75 w100] -> w69
      tunnel: w70 -> [_ w90]
      tunnel: [w74 w98] -> w68
      tunnel: w66 -> [w74 w96]
      tunnel: w62 -> [_ _]
      tunnel: [_ w95] -> w60
      tunnel: [_ w80] -> w59
      tunnel: w58 -> [_ w91]
      tunnel: w57 -> [_ _]
      tunnel: w56 -> [_ _]
      tunnel: w55 -> [w73 w89]
      tunnel: [w73 w87] -> w54
      tunnel: w53 -> [w72 w76]
      tunnel: [w72 w76] -> w52
      frame 0, Default {
        # "No arrays modified.\nPass them on as is."
      }
      frame 8 {
        # "Modify specified fields for 87 Sr Arbitrary\nWaveforms array and create array\nof arrays to pass along to higher\nlevel VI. (87Sr Red MOT Waveform)"
        n13 = Unbundle(w91) -> ("Channel to Change"=w94:i8, "Interval to Change"=w93:i8, "Waveform Parameter\nto Change"=w92:u16)
        n14 = case shown="6" w92 {
          tunnel: w102 -> [w121 w139 w155 w172 w189 w206 w223 w240 w255]
          tunnel: w94 -> [w115 w138 w154 w171 w188 w205 w222 w239 _]
          tunnel: w93 -> [w120 w137 w153 w170 w187 w204 w221 w238 w253]
          tunnel: w101 -> [w116 w133 w149 w166 w183 w200 w217 w234 w251]
          tunnel: [w118 w135 w151 w168 w185 w202 w219 w236 w255] -> w100
          tunnel: w96 -> [w117 w134 w150 w167 w184 w201 w218 w235 w254]
          tunnel: [w117 w134 w150 w167 w184 w201 w218 w235 w252] -> w98
          tunnel: [w116 w133 w149 w166 w183 w200 w217 w234 w251] -> w95
          tunnel: [FALSE FALSE FALSE FALSE FALSE FALSE FALSE FALSE TRUE] -> _
          frame 0, Default {
            # "Change constant"
            n15 = Index Array(array=w121, index (row)=w115, index (col)=w120) -> (element=w130:T10)
            n16 = Unbundle(w130) -> ("AC Frequency (kHz)"=w129:dbl, "Initial AC Ampl. (p-p/2)"=w128:dbl, "Final AC Ampl."=w127:dbl, "Initial DC Value"=w126:dbl, "Final DC Value"=w125:dbl, "Gamma AC"=w124:dbl, "String"=w122:string, "Gamma DC"=w123:dbl)  [unwired: 1 out]
            n17 = Bundle(cluster=w130, "AC Frequency (kHz)"=w129, "Initial AC Ampl. (p-p/2)"=w128, "Final AC Ampl."=w127, "Initial DC Value"=w126, "Final DC Value"=w125, "Constant"=w116, "Gamma AC"=w124, "String"=w122, "Gamma DC"=w123) -> (w119:T10)
            n18 = Replace Array Subset(array=w121, new element=w119, index (row)=w115, index (col)=w120) -> (w118:T2)
          }
          frame 1 {
            # "Change Initial DC"
            n19 = Index Array(array=w139, index (row)=w138, index (col)=w137) -> (element=w147:T10)
            n20 = Unbundle(w147) -> ("AC Frequency (kHz)"=w146:dbl, "Initial AC Ampl. (p-p/2)"=w145:dbl, "Final AC Ampl."=w144:dbl, "Final DC Value"=w132:dbl, "Constant"=w143:dbl, "Gamma AC"=w142:dbl, "String"=w140:string, "Gamma DC"=w141:dbl)  [unwired: 1 out]
            n21 = Bundle(cluster=w147, "AC Frequency (kHz)"=w146, "Initial AC Ampl. (p-p/2)"=w145, "Final AC Ampl."=w144, "Initial DC Value"=w133, "Final DC Value"=w132, "Constant"=w143, "Gamma AC"=w142, "String"=w140, "Gamma DC"=w141) -> (w136:T10)
            n22 = Replace Array Subset(array=w139, new element=w136, index (row)=w138, index (col)=w137) -> (w135:T2)
          }
          frame 2 {
            # "Change Final DC"
            n23 = Index Array(array=w155, index (row)=w154, index (col)=w153) -> (element=w164:T10)
            n24 = Unbundle(w164) -> ("AC Frequency (kHz)"=w163:dbl, "Initial AC Ampl. (p-p/2)"=w162:dbl, "Final AC Ampl."=w161:dbl, "Initial DC Value"=w160:dbl, "Constant"=w159:dbl, "Gamma AC"=w158:dbl, "String"=w156:string, "Gamma DC"=w157:dbl)  [unwired: 1 out]
            n25 = Bundle(cluster=w164, "AC Frequency (kHz)"=w163, "Initial AC Ampl. (p-p/2)"=w162, "Final AC Ampl."=w161, "Initial DC Value"=w160, "Final DC Value"=w149, "Constant"=w159, "Gamma AC"=w158, "String"=w156, "Gamma DC"=w157) -> (w152:T10)
            n26 = Replace Array Subset(array=w155, new element=w152, index (row)=w154, index (col)=w153) -> (w151:T2)
          }
          frame 3 {
            # "Change Gamma DC"
            n27 = Index Array(array=w172, index (row)=w171, index (col)=w170) -> (element=w181:T10)
            n28 = Unbundle(w181) -> ("AC Frequency (kHz)"=w180:dbl, "Initial AC Ampl. (p-p/2)"=w179:dbl, "Final AC Ampl."=w178:dbl, "Initial DC Value"=w177:dbl, "Final DC Value"=w176:dbl, "Constant"=w175:dbl, "Gamma AC"=w174:dbl, "String"=w173:string)  [unwired: 1 out]
            n29 = Bundle(cluster=w181, "AC Frequency (kHz)"=w180, "Initial AC Ampl. (p-p/2)"=w179, "Final AC Ampl."=w178, "Initial DC Value"=w177, "Final DC Value"=w176, "Constant"=w175, "Gamma AC"=w174, "String"=w173, "Gamma DC"=w166) -> (w169:T10)
            n30 = Replace Array Subset(array=w172, new element=w169, index (row)=w171, index (col)=w170) -> (w168:T2)
          }
          frame 4 {
            # "Change AC Freq."
            n31 = Index Array(array=w189, index (row)=w188, index (col)=w187) -> (element=w198:T10)
            n32 = Unbundle(w198) -> ("Initial AC Ampl. (p-p/2)"=w197:dbl, "Final AC Ampl."=w196:dbl, "Initial DC Value"=w195:dbl, "Final DC Value"=w194:dbl, "Constant"=w193:dbl, "Gamma AC"=w192:dbl, "String"=w190:string, "Gamma DC"=w191:dbl)  [unwired: 1 out]
            n33 = Bundle(cluster=w198, "AC Frequency (kHz)"=w183, "Initial AC Ampl. (p-p/2)"=w197, "Final AC Ampl."=w196, "Initial DC Value"=w195, "Final DC Value"=w194, "Constant"=w193, "Gamma AC"=w192, "String"=w190, "Gamma DC"=w191) -> (w186:T10)
            n34 = Replace Array Subset(array=w189, new element=w186, index (row)=w188, index (col)=w187) -> (w185:T2)
          }
          frame 5 {
            # "Change Initial AC"
            n35 = Index Array(array=w206, index (row)=w205, index (col)=w204) -> (element=w215:T10)
            n36 = Unbundle(w215) -> ("AC Frequency (kHz)"=w214:dbl, "Final AC Ampl."=w213:dbl, "Initial DC Value"=w212:dbl, "Final DC Value"=w211:dbl, "Constant"=w210:dbl, "Gamma AC"=w209:dbl, "String"=w207:string, "Gamma DC"=w208:dbl)  [unwired: 1 out]
            n37 = Bundle(cluster=w215, "AC Frequency (kHz)"=w214, "Initial AC Ampl. (p-p/2)"=w200, "Final AC Ampl."=w213, "Initial DC Value"=w212, "Final DC Value"=w211, "Constant"=w210, "Gamma AC"=w209, "String"=w207, "Gamma DC"=w208) -> (w203:T10)
            n38 = Replace Array Subset(array=w206, new element=w203, index (row)=w205, index (col)=w204) -> (w202:T2)
          }
          frame 6 {
            # "Change Final AC"
            n39 = Index Array(array=w223, index (row)=w222, index (col)=w221) -> (element=w232:T10)
            n40 = Unbundle(w232) -> ("AC Frequency (kHz)"=w231:dbl, "Initial AC Ampl. (p-p/2)"=w230:dbl, "Initial DC Value"=w229:dbl, "Final DC Value"=w228:dbl, "Constant"=w227:dbl, "Gamma AC"=w226:dbl, "String"=w224:string, "Gamma DC"=w225:dbl)  [unwired: 1 out]
            n41 = Bundle(cluster=w232, "AC Frequency (kHz)"=w231, "Initial AC Ampl. (p-p/2)"=w230, "Final AC Ampl."=w217, "Initial DC Value"=w229, "Final DC Value"=w228, "Constant"=w227, "Gamma AC"=w226, "String"=w224, "Gamma DC"=w225) -> (w220:T10)
            n42 = Replace Array Subset(array=w223, new element=w220, index (row)=w222, index (col)=w221) -> (w219:T2)
          }
          frame 7 {
            # "Change Gamma AC"
            n43 = Index Array(array=w240, index (row)=w239, index (col)=w238) -> (element=w249:T10)
            n44 = Unbundle(w249) -> ("AC Frequency (kHz)"=w248:dbl, "Initial AC Ampl. (p-p/2)"=w247:dbl, "Final AC Ampl."=w246:dbl, "Initial DC Value"=w245:dbl, "Final DC Value"=w244:dbl, "Constant"=w243:dbl, "String"=w241:string, "Gamma DC"=w242:dbl)  [unwired: 1 out]
            n45 = Bundle(cluster=w249, "AC Frequency (kHz)"=w248, "Initial AC Ampl. (p-p/2)"=w247, "Final AC Ampl."=w246, "Initial DC Value"=w245, "Final DC Value"=w244, "Constant"=w243, "Gamma AC"=w234, "String"=w241, "Gamma DC"=w242) -> (w237:T10)
            n46 = Replace Array Subset(array=w240, new element=w237, index (row)=w239, index (col)=w238) -> (w236:T2)
          }
          frame 8 {
            # "Change Time Interval"
            n47 = Replace Array Subset(array=w254, new element=w251, index=w253) -> (w252:dbl[])
          }
        }
        n48 = for {
          tunnel: w98 -> [w107] mode=indexing
          tunnel: w90 -> [w109] mode=indexing
          shift-right: [w106] -> w99
          shift-left: 0.0 -> [w108]
          n49 = case shown="True" w109 {
            tunnel: w108 -> [w110 w113]
            tunnel: w107 -> [_ w112]
            tunnel: [w110 w111] -> w106
            frame False {
              # "zero s"
            }
            frame True {
              n50 = Add(x=w112, y=w113) -> (x+y=w111:dbl)
            }
          }
        }
        n51 = Index Array(array=w89, index=w88) -> (element=w79:T11)
        n52 = Unbundle By Name(w79) -> ("Data Field"=w83:u32, "Output Bits"=w84:bool[], "Delay"=w82:dbl, "String"=w86:string, "OP code"=w85:u8)
        n53 = Divide(x=w99, y=1000) -> (x/y=w80:dbl)
        n54 = case shown="True" "Case Constant\n(See Context Help)" {
          tunnel: w82 -> [w104 _]
          tunnel: [w104 w105] -> w81
          tunnel: w80 -> [_ w105]
          frame False {
            # "no \nchange"
          }
          frame True {
            # "match \nintervals"
          }
        }
        n55 = Bundle By Name(cluster=w79, "Data Field"=w83, "Output Bits"=w84, "Delay"=w81, "String"=w86, "OP code"=w85) -> (w78:T11)
        n56 = Replace Array Subset(array=w89, new element=w78, index=w88) -> (w87:T4)
      }
    }
  }
  "87 Sr ArbWaveform \nArray of Channels" <- w41
  "87Sr ArbWaveform Interval Lengths" <- w40
  "changed\nquantity" <- w22
  "red mot cooling time" <- w20
  "PB Array of Arrays" <- w3
  "Lattice Waveform \nArray of Channels" <- w1
  n57 = Bundle("PB parameter to change"=w33, "Column of\nData to Change\n(0, 1, 2, ....)"=w32, "Column of\nDelay to Change\n(0, 1, 2, ....)"=w31, "6713 DAC Ch\nto Change"=w30, "column for waveform\n(red mot cooling)"=w28, "column for waveform\n(dipole trap loading)"=w16) -> (→"output params to change":T8)  [unwired: 1 in]
